vi "color_sensor_old.vi"() -> ()   [LabVIEW 2022 SP3]
uses:
  <vilib>/DAQmx/write.llb/DAQmx Write (Digital Bool 1Line 1Point).vi
  <vilib>/DAQmx/create/channels.llb/DAQmx Create Channel (DO-Digital Output).vi
  <vilib>/DAQmx/miscellaneous.llb/DAQmx Fill In Error Info.vi
  <vilib>/Instr/_visa.llb/VISA Configure Serial Port (Instr).vi
panel:
  in  "VISA resource name":refnum<visa-resource-name>
  in  "stop 2":bool
  out "read buffer":string
  in  "Blue Channel":tag
  in  "Green Channel":tag
  in  "Red Channel":tag
  in  "stop":bool
  out "green":bool
  out "blue":bool
  out "red":bool
  out "Numeric":i32
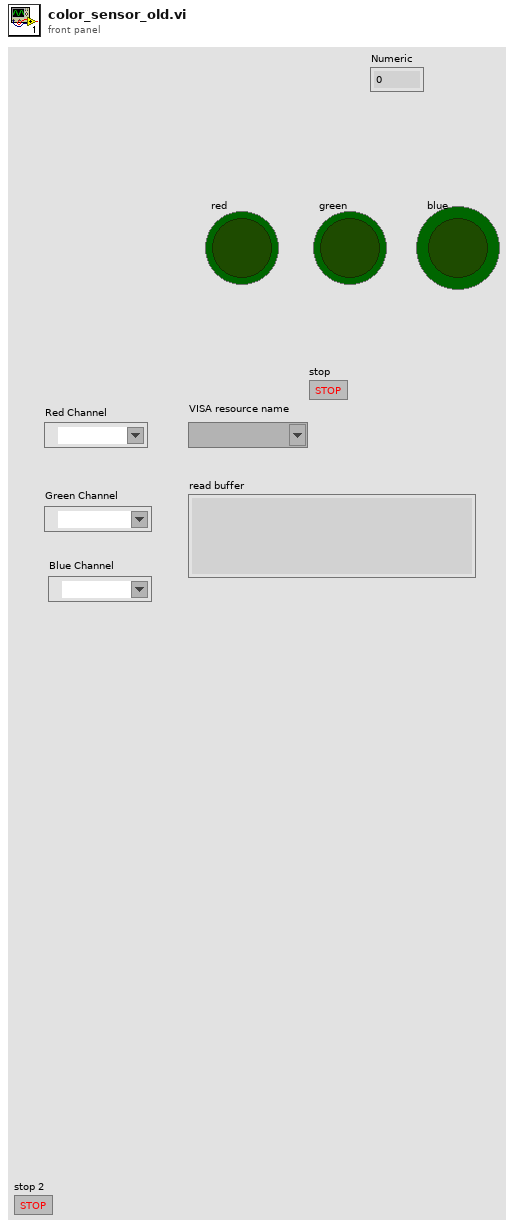
[diagram p1: front panel]
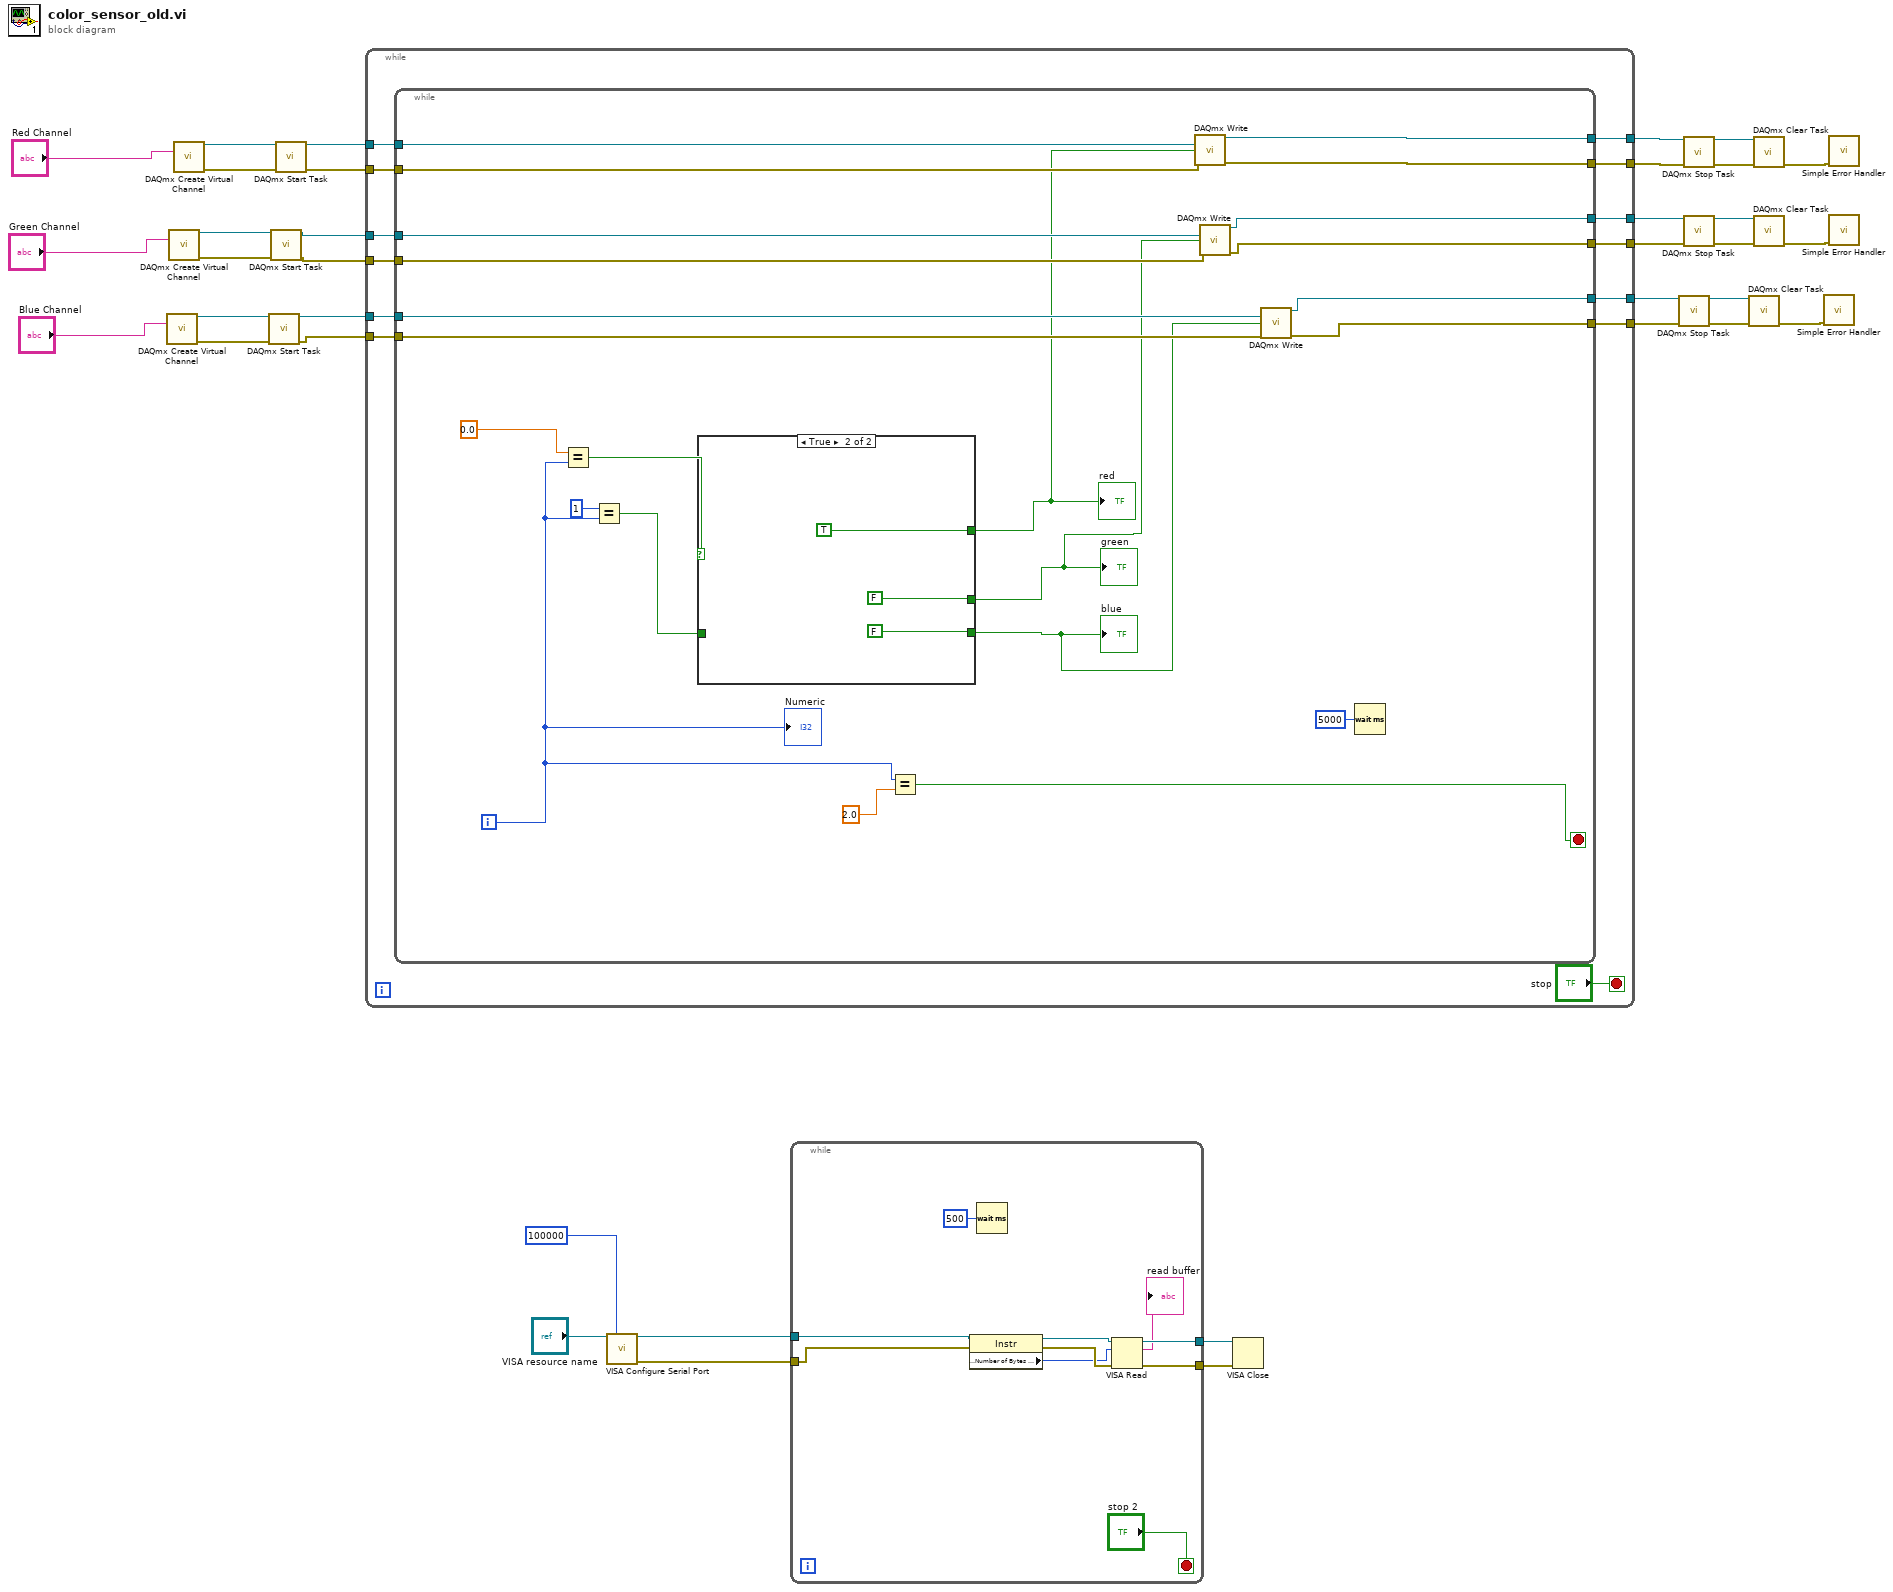
[diagram p0: block diagram]
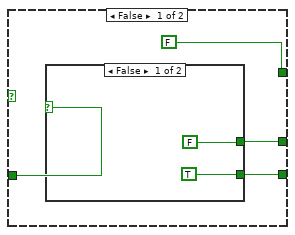
[diagram p2: hidden frame]
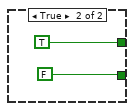
[diagram p3: hidden frame]
diagram:
  n1 = call-poly <vilib>:"DAQmx Create Virtual Channel.vi"("lines"="Blue Channel") -> ("task out"=w17:refnum<k21>, "error out"=w18:errorcluster)  [unwired: 13 in]
  n2 = call-poly <vilib>:"DAQmx Create Virtual Channel.vi"("lines"="Green Channel") -> ("task out"=w26:refnum<k21>, "error out"=w27:errorcluster)  [unwired: 13 in]
  n3 = call-poly <vilib>:"DAQmx Create Virtual Channel.vi"("lines"="Red Channel") -> ("task out"=w35:refnum<k21>, "error out"=w36:errorcluster)  [unwired: 13 in]
  n4 = call <vilib>:"DAQmx Start Task.vi"("task/channels in"=w17, "error in"=w18) -> ("task out"=w16:refnum<k21>, "error out"=w15:errorcluster)  [unwired: 12 in]
  n5 = call <vilib>:"DAQmx Start Task.vi"("task/channels in"=w26, "error in"=w27) -> ("task out"=w25:refnum<k21>, "error out"=w24:errorcluster)  [unwired: 12 in]
  n6 = call <vilib>:"DAQmx Start Task.vi"("task/channels in"=w35, "error in"=w36) -> ("task out"=w34:refnum<k21>, "error out"=w33:errorcluster)  [unwired: 12 in]
  n7 = while {
    tunnel: w34 -> [w48]
    tunnel: w33 -> [w47]
    tunnel: [w46] -> w29
    tunnel: [w45] -> w28
    tunnel: w25 -> [w44]
    tunnel: w24 -> [w43]
    tunnel: [w42] -> w20
    tunnel: [w41] -> w19
    tunnel: w16 -> [w40]
    tunnel: w15 -> [w39]
    tunnel: [w38] -> w11
    tunnel: [w37] -> w10
    stop <- "stop" stop-if-true
    n8 = while {
      tunnel: w48 -> [w64]
      tunnel: w47 -> [w63]
      tunnel: [w62] -> w46
      tunnel: [w61] -> w45
      tunnel: w44 -> [w60]
      tunnel: w43 -> [w59]
      tunnel: [w58] -> w42
      tunnel: [w57] -> w41
      tunnel: w40 -> [w56]
      tunnel: w39 -> [w55]
      tunnel: [w54] -> w38
      tunnel: [w53] -> w37
      i -> [w66]
      stop <- w71 stop-if-true
      n9 = Equal?(x=0.0, y=w66) -> (x = y?=w68:bool)
      n10 = Equal?(x=1, y=w66) -> (x = y?=w67:bool)
      n11 = case shown="True" w68 {
        tunnel: [FALSE TRUE] -> w52
        tunnel: w67 -> [w76 _]
        tunnel: [w74 FALSE] -> w51
        tunnel: [w73 FALSE] -> w50
        frame False {
          n12 = case shown="False" w76 {
            tunnel: [FALSE TRUE] -> w74
            tunnel: [TRUE FALSE] -> w73
            frame False {
            }
            frame True {
            }
          }
        }
        frame True {
        }
      }
      "red" <- w52
      "blue" <- w50
      "green" <- w51
      n13 = Equal?(x=w66, y=2.0) -> (x = y?=w71:bool)
      n14 = call-poly <vilib>:"DAQmx Write.vi"("task/channels in"=w64, "data"=w52, "error in"=w63) -> ("task out"=w62:refnum<k21>, "error out"=w61:errorcluster)  [unwired: 10 in, 1 out]
      n15 = call-poly <vilib>:"DAQmx Write.vi"("task/channels in"=w60, "data"=w51, "error in"=w59) -> ("task out"=w58:refnum<k21>, "error out"=w57:errorcluster)  [unwired: 10 in, 1 out]
      n16 = call-poly <vilib>:"DAQmx Write.vi"("task/channels in"=w56, "data"=w50, "error in"=w55) -> ("task out"=w54:refnum<k21>, "error out"=w53:errorcluster)  [unwired: 10 in, 1 out]
      n17 = Wait (ms)(milliseconds to wait=u32 5000) -> ()  [unwired: 1 out]
      "Numeric" <- w66
    }
  }
  n18 = call-poly "VISA Configure Serial Port"("VISA resource name"="VISA resource name", "timeout (10sec)"=u32 100000) -> ("VISA resource name out"=w4:refnum<visa-resource-name>, "error out"=w3:errorcluster)  [unwired: 12 in]
  n19 = while {
    tunnel: w4 -> [w85]
    tunnel: w3 -> [w84]
    tunnel: [w90] -> w2
    tunnel: [w89] -> w1
    stop <- "stop 2" stop-if-true
    n20 = property class="Instr"(reference=w85, error in=w84) -> (reference out=w93:refnum<visa-resource-name>, error out=w92:errorcluster, "Serial Settings:Number of Bytes at Serial Port"=w91:u32)
    n21 = Wait (ms)(milliseconds to wait=u32 500) -> ()  [unwired: 1 out]
    n22 = VISA Read(VISA resource name=w93, byte count=w91, error in (no error)=w92) -> (VISA resource name out=w90:refnum<visa-resource-name>, read buffer=→"read buffer":string, error out=w89:errorcluster)  [unwired: 1 out]
  }
  n23 = VISA Close(VISA resource name=w2, error in (no error)=w1) -> ()  [unwired: 1 out]
  n24 = call <vilib>:"DAQmx Stop Task.vi"("task/channels in"=w11, "error in"=w10) -> ("task out"=w14:refnum<k21>, "error out"=w13:errorcluster)  [unwired: 12 in]
  n25 = call <vilib>:"DAQmx Stop Task.vi"("task/channels in"=w29, "error in"=w28) -> ("task out"=w32:refnum<k21>, "error out"=w31:errorcluster)  [unwired: 12 in]
  n26 = call <vilib>:"DAQmx Stop Task.vi"("task/channels in"=w20, "error in"=w19) -> ("task out"=w23:refnum<k21>, "error out"=w22:errorcluster)  [unwired: 12 in]
  n27 = call <vilib>:"DAQmx Clear Task.vi"("task in"=w14, "error in"=w13) -> ("error out"=w12:errorcluster)  [unwired: 13 in]
  n28 = call <vilib>:"DAQmx Clear Task.vi"("task in"=w32, "error in"=w31) -> ("error out"=w30:errorcluster)  [unwired: 13 in]
  n29 = call <vilib>:"DAQmx Clear Task.vi"("task in"=w23, "error in"=w22) -> ("error out"=w21:errorcluster)  [unwired: 13 in]
  n30 = call <vilib>:"Simple Error Handler.vi"("error in (no error)"=w12) -> ()  [unwired: 4 in, 5 out]
  n31 = call <vilib>:"Simple Error Handler.vi"("error in (no error)"=w30) -> ()  [unwired: 4 in, 5 out]
  n32 = call <vilib>:"Simple Error Handler.vi"("error in (no error)"=w21) -> ()  [unwired: 4 in, 5 out]
